vi "未命名 4.vi"() -> ()   [LabVIEW 2016]
uses:
  Espresso/Espresso.lvclass
  CondimentDecorator/Mocha/Mocha.lvclass
panel:
  out "Cost":dbl
  out "Description":string
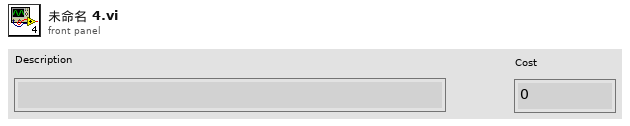
[diagram p1: front panel]
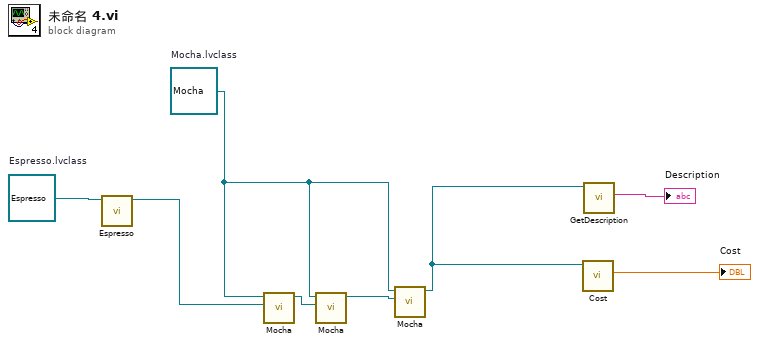
[diagram p0: block diagram]
diagram:
  w2 = refnum<class "Mocha.lvclass"> refnum  # Mocha.lvclass
  w8 = refnum<class "Espresso.lvclass"> refnum  # Espresso.lvclass
  n1 = call "Espresso.vi"("Espresso 输入"=w8) -> ("Espresso 输出"=w5:refnum<class "Espresso.lvclass">)  [unwired: 9 in, 1 out]
  n2 = call "Mocha.vi"("Beverage.lvclass"=w5, "Mocha 输入"=w2) -> ("Mocha 输出"=w1:refnum<class "Mocha.lvclass">)  [unwired: 8 in, 1 out]
  n3 = call "Mocha.vi"("Beverage.lvclass"=w1, "Mocha 输入"=w2) -> ("Mocha 输出"=w3:refnum<class "Mocha.lvclass">)  [unwired: 8 in, 1 out]
  n4 = call "Mocha.vi"("Beverage.lvclass"=w3, "Mocha 输入"=w2) -> ("Mocha 输出"=w4:refnum<class "Mocha.lvclass">)  [unwired: 8 in, 1 out]
  n5 = call-dynamic "Cost.vi"("Mocha 输入"=w4) -> ("Cost"=→"Cost":dbl)  [unwired: 8 in, 2 out]
  n6 = call-dynamic "GetDescription.vi"("Mocha 输入"=w4) -> ("Description"=→"Description":string)  [unwired: 8 in, 2 out]
